vi "Restart.SaveSettings.vi"(8 "error in":errorcluster, 10 "Restart Settings":T1={"LogFile"=path "", "Log Settings"=[], "StimulusProfile"=path "", "StopIteration"=0, "StopStep"=0, "Log Channels"=enum."Aliases", "Base File Name"="Log", "Enable Logging"=TRUE, "Profile"="", "StopDuration"=0.0, "Waveform Definition"=path "", "Number of Cycles"=0.0, "Cyclic Frequency"=0.0, "Work Order Number"="", "Operator Name"="", "Description"="", "Station.ID"="", "Sequence.Channels"=[], "Alarms"=[]} {"Alarms"."Delay" format="%.2f"; "Alarms"."Low Limit" format="%.2f"; "Alarms"."High Limit" format="%.2f"}, 11 "datalog path (use dialog)":path) -> (0 "error out":errorcluster, 3 "path":path)   [LabVIEW 2015, in "Single Station Execution.lvlib"]
uses:
  Single Station Execution.lvlib
  Types/Restart.Settings.ctl
  <vilib>/NI Veristand/Execution/DataLogging/TDMS Channel Group.ctl
  <vilib>/NI Veristand/Execution/DataLogging/TDMS Property.ctl
  <vilib>/NI Veristand/Execution/DataLogging/TDMS Channel.ctl
  <vilib>/NI Veristand/Execution/DataLogging/Time Channel Options.ctl
  Types/Log.SelectedChannels.ctl
  Types/Config.AlarmSettings.ctl
  Main.Constants.vi
  <vilib>/NI/GXML/GXML.lvlib
  <vilib>/NI Veristand/Execution/DataLogging/NI_VS Data Logging API.lvlib
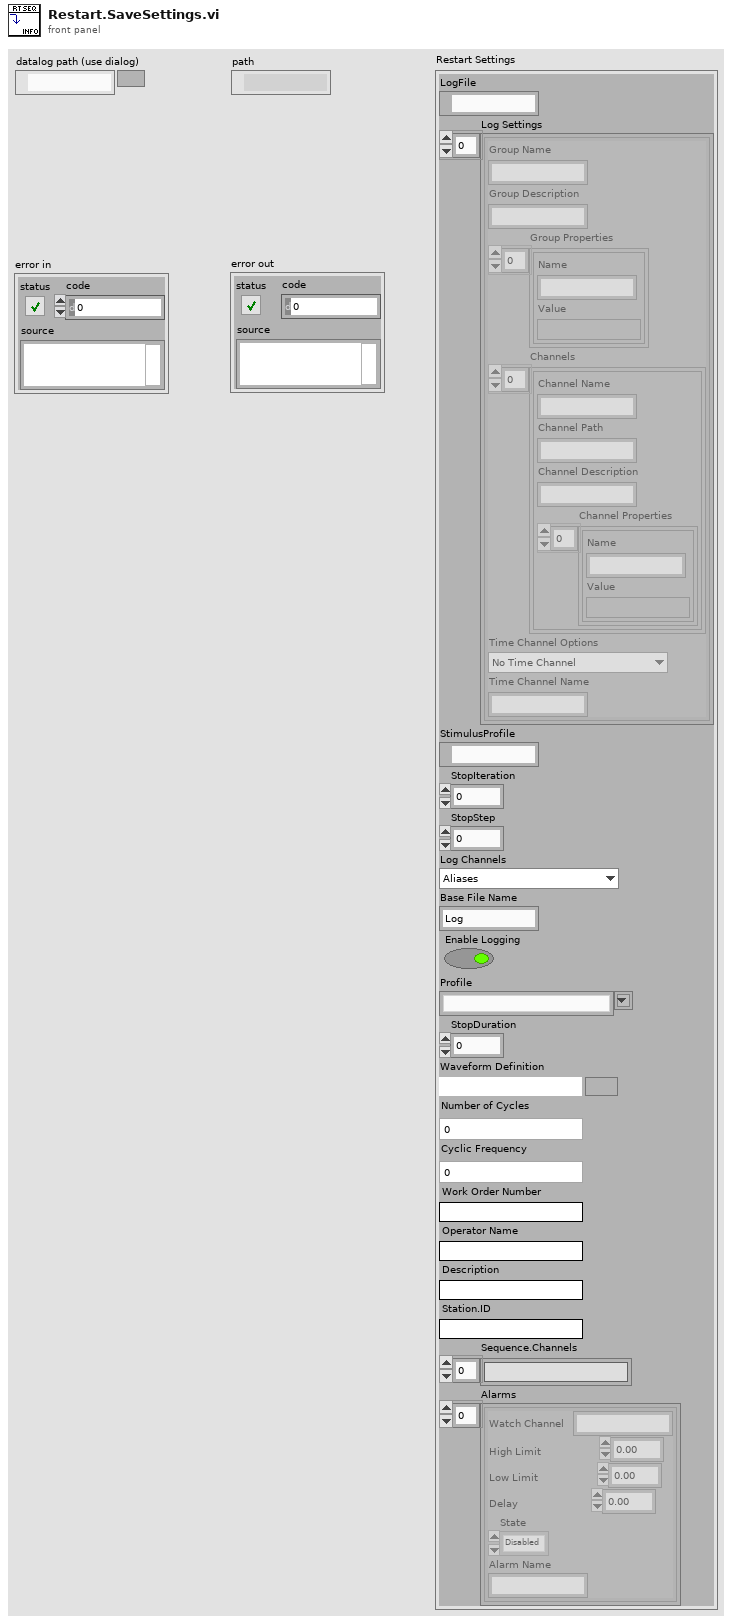
[diagram p1: front panel]
types:
  T1 = typedef "Single Station Execution.lvlib/Restart.Settings.ctl" = cluster{"LogFile":path, "Log Settings":T2[], "StimulusProfile":path, "StopIteration":u32, "StopStep":u32, "Log Channels":T6, "Base File Name":string, "Enable Logging":bool, "Profile":string, "StopDuration":dbl, "Waveform Definition":path, "Number of Cycles":dbl, "Cyclic Frequency":dbl, "Work Order Number":string, "Operator Name":string, "Description":string, "Station.ID":string, "Sequence.Channels":string[], "Alarms":T7[]}
  T2 = typedef "NI_VS Data Logging API.lvlib/TDMS Channel Group.ctl" = cluster{"Group Name":string, "Group Description":string, "Group Properties":T3[], "Channels":T4[], "Time Channel Options":T5, "Time Channel Name":string}
  T3 = typedef "NI_VS Data Logging API.lvlib/TDMS Property.ctl" = cluster{"Name":string, "Value":variant}
  T4 = typedef "NI_VS Data Logging API.lvlib/TDMS Channel.ctl" = cluster{"Channel Name":string, "Channel Path":string, "Channel Description":string, "Channel Properties":T3[]}
  T5 = typedef "NI_VS Data Logging API.lvlib/Time Channel Options.ctl" = enum16{"No Time Channel", "Absolute Time", "System Time", "System Time - Microseconds", "Absolute Time as Double"}
  T6 = typedef "Single Station Execution.lvlib/Log.SelectedChannels.ctl" = enum16{"Channels (No System Channel)", "Aliases", "All"}
  T7 = typedef "Single Station Execution.lvlib/Config.AlarmSettings.ctl" = cluster{"Watch Channel":string, "High Limit":dbl, "Low Limit":dbl, "Delay":dbl, "State":enum16{"Disabled", "Enabled", "Tripped", "Delayed Trip", "Indicate"}, "Alarm Name":string}
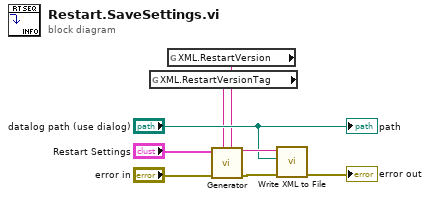
[diagram p0: block diagram]
diagram:
  n1 = global read "Main.Constants.vi" "XML.RestartVersionTag"() -> (w2:string)
  n2 = global read "Main.Constants.vi" "XML.RestartVersion"() -> (w1:string)
  n3 = call <vilib>:"Generator.vi"("Version String"=w1, "Version Tag Name"=w2, "error in"="error in", "Variant"="Restart Settings") -> ("error out"=w7:errorcluster, "XML String Out"=w8:string)  [unwired: 6 in]
  n4 = call <vilib>:"Write XML to File.vi"("error in"=w7, "XML File Path"="datalog path (use dialog)", "XML Input"=w8) -> ("error out"=→"error out":errorcluster)  [unwired: 8 in]
  "path" <- "datalog path (use dialog)"
